vi "Initialize.vi"(8 "error in (no error)":errorcluster, 10 "Device":string) -> (0 "error out":errorcluster, 3 "DigitalIO out":refnum<class "DigitalIO.lvclass">)   [LabVIEW 2018, in "DigitalIO.lvlib" / "DigitalIO.lvclass"]
uses:
  DigitalIO.lvclass
  DigitalIO.lvclass/DigitalIO.ctl
  PPLs/Configuration/Configuration.lvlibp/Configuration.lvclass
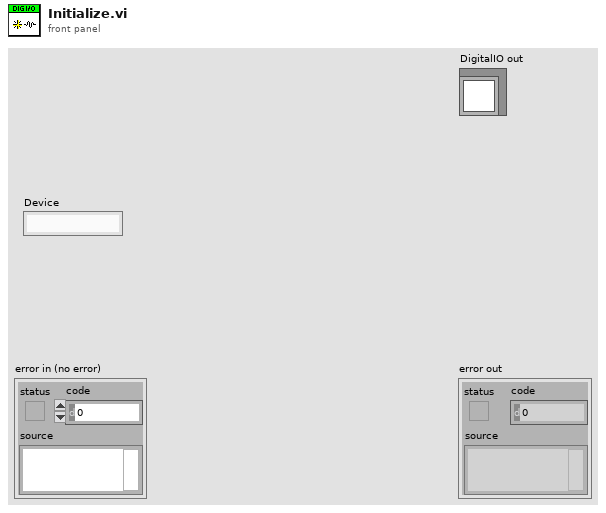
[diagram p1: front panel]
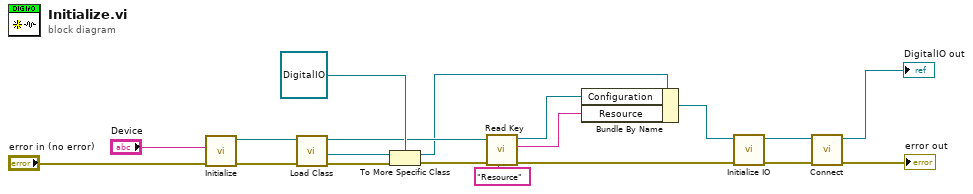
[diagram p0: block diagram]
diagram:
  n1 = call "Initialize.vi"("error in"="error in (no error)", "Device"="Device") -> ("error out"=w16:errorcluster, "Configuration out"=w17:refnum<class "Configuration.lvclass">)  [unwired: 8 in]
  n2 = call "Load Class.vi"("error in"=w16, "Configuration in"=w17) -> ("error out"=w15:errorcluster, "Class out"=w14:refnum<class>, "Configuration out"=w11:refnum<class "Configuration.lvclass">)  [unwired: 7 in]
  n3 = To More Specific Class(target class=refnum<class "DigitalIO.lvclass"> refnum ("DigitalIO in"), reference=w14, error in=w15) -> (specific class reference=w9:refnum<class "DigitalIO.lvclass">, error out=w12:errorcluster)
  n4 = call "Read Key.vi"("Key:"="Resource", "error in"=w12, "Configuration in"=w11) -> ("error out"=w2:errorcluster, "Value"=w7:string, "Configuration out"=w8:refnum<class "Configuration.lvclass">)  [unwired: 6 in]
  n5 = Bundle By Name(cluster=w9, "Configuration"=w8, "Resource"=w7) -> (w4:refnum<class "DigitalIO.lvclass">)
  n6 = call "Initialize IO.vi"("error in (no error)"=w2, "DigitalIO in"=w4) -> ("error out"=w1:errorcluster, "DigitalIO out"=w3:refnum<class "DigitalIO.lvclass">)  [unwired: 8 in]
  n7 = call-dynamic "Connect.vi"("error in (no error)"=w1, "DigitalIO in"=w3) -> ("error out"=→"error out":errorcluster, "DigitalIO out"=→"DigitalIO out":refnum<class "DigitalIO.lvclass">)  [unwired: 8 in]
